vi "Write Results Manager.vi"(8 "error in (no error)":errorcluster, 10 "Results Manager.lvclass":refnum<class "Results Manager.lvclass">, 11 "Sequence Engine in":refnum<class "Sequence Engine.lvclass">) -> (0 "error out":errorcluster, 3 "Sequence Engine out":refnum<class "Sequence Engine.lvclass">)   [LabVIEW 2021, in "Sequence Engine.lvlib" / "Sequence Engine.lvclass"]
uses:
  Sequence Engine.lvclass
  Results Manager/Results Manager.lvclass
  Sequence Engine.lvclass/Sequence Engine.ctl
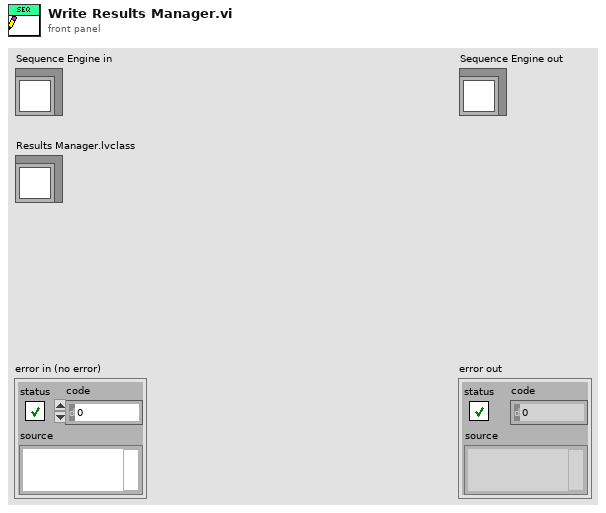
[diagram p1: front panel]
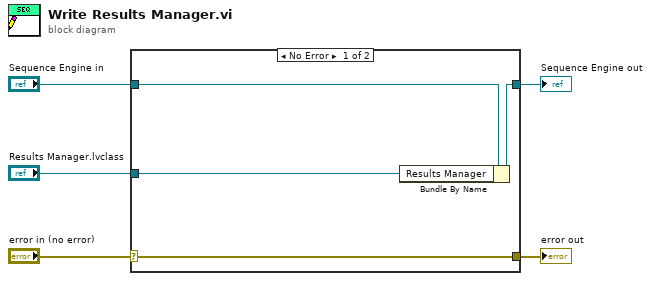
[diagram p0: block diagram]
diagram:
  n1 = case shown="No Error" "error in (no error)" {
    selector: "error in (no error)" -> [w9 w10]
    tunnel: [w9 w10] -> w4
    tunnel: [w7 w11] -> w2
    tunnel: "Sequence Engine in" -> [w8 w11]
    tunnel: "Results Manager.lvclass" -> [w6 _]
    frame No Error {
      n2 = Bundle By Name(cluster=w8, "Results Manager"=w6) -> (w7:refnum<class "Sequence Engine.lvclass">)
    }
    frame Error {
    }
  }
  "error out" <- w4
  "Sequence Engine out" <- w2
